vi "Read Measurement Result.vi"   [LabVIEW 2023, in "Agilent B2900 Series.lvlib"]
doc: "Read the measurement result of current, voltage or resistance measurement"
uses:
  Agilent B2900 Series.lvlib
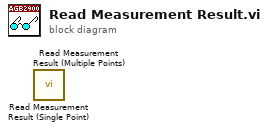
[diagram p0: block diagram]
diagram:
  n1 = call "Read Measurement Result (Single Point).vi"() -> ()  [unwired: 9 in, 3 out]
  n2 = call "Read Measurement Result (Multiple Points).vi"() -> ()  [unwired: 9 in, 3 out]
